vi "getProperty.vi"(8 "error in (no error)":errorcluster, 10 "Property Name in":string, 11 "IPropertyObject in":refnum<class "IPropertyObject.lvclass">) -> (0 "error out":errorcluster, 2 "Property out":refnum<class "IProperty.lvclass">, 3 "IPropertyObject out":refnum<class "IPropertyObject.lvclass">)   [LabVIEW 2022 SP3, in "openDAQ.lvlib" / "IBaseObject.lvlib" / "IPropertyObject.lvlib" / "IPropertyObject.lvclass"]
uses:
  <instrlib>/openDAQ/Public/Classes/IPropertyObject/IPropertyObject.lvclass
  <instrlib>/openDAQ/Public/Classes/IPropertyObject/IPropertyObject.lvclass/IPropertyObject.ctl
  <instrlib>/openDAQ/Public/Classes/daqCoreTypes/IString/IString.lvclass
  <instrlib>/openDAQ/Public/Classes/IProperty/IProperty.lvclass
  <instrlib>/openDAQ/Binaries/Windows/x86/copendaq32.dll
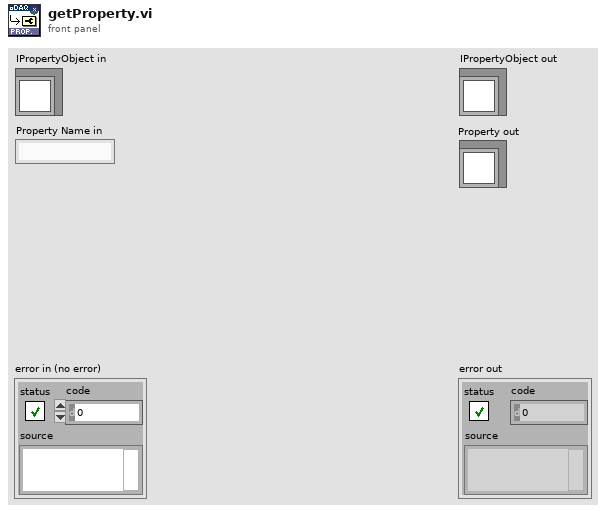
[diagram p1: front panel]
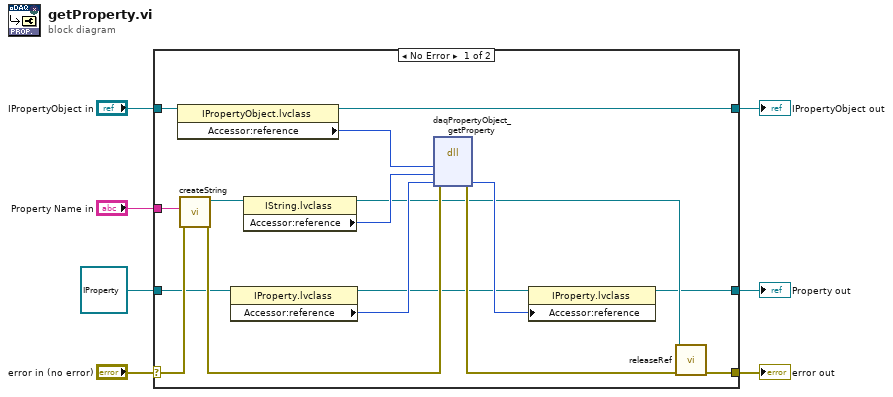
[diagram p0: block diagram]
diagram:
  n1 = case shown="No Error" "error in (no error)" {
    selector: "error in (no error)" -> [w18 w26]
    tunnel: [w13 w26] -> w6
    tunnel: [w19 w25] -> w4
    tunnel: "IPropertyObject in" -> [w21 w25]
    tunnel: "Property Name in" -> [w16 _]
    tunnel: refnum<class "IProperty.lvclass"> refnum ("openDAQ.lvlib:IBaseObject.lvlib:IProperty.lvlib:IProperty.lvclass") -> [w10 w24]
    tunnel: [w8 w24] -> w1
    frame No Error {
      n2 = property class="IPropertyObject.lvclass"(reference=w21) -> (reference out=w19:refnum<class "IPropertyObject.lvclass">, "Accessor:reference"=w20:i64)  [unwired: 1 in, 1 out]
      n3 = call <instrlib>:"createString.vi"("error in (no error)"=w18, "String"=w16) -> ("error out"=w17:errorcluster, "IString out"=w15:refnum<class "IString.lvclass">)  [unwired: 8 in]
      n4 = property class="IProperty.lvclass"(reference=w10) -> (reference out=w9:refnum<class "IProperty.lvclass">, "Accessor:reference"=w22:i64)  [unwired: 1 in, 1 out]
      n5 = property class="IString.lvclass"(reference=w15) -> (reference out=w11:refnum<class "IString.lvclass">, "Accessor:reference"=w14:i64)  [unwired: 1 in, 1 out]
      n6 = dll-call lib="C:/Program Files (x86)/National Instruments/LabVIEW 2022/instr.lib/openDAQ/Binaries/Windows/x86/copendaq*.*" fn="daqPropertyObject_getProperty"(error in=w17, "propertyObject"=w20, "name"=w14, "hasProperty"=w22) -> (error out=w12:errorcluster, "hasProperty"=w23:i64)  [unwired: 5 in, 1 out]
      n7 = property class="IProperty.lvclass"(reference=w9, "Accessor:reference"=w23) -> (reference out=w8:refnum<class "IProperty.lvclass">)  [unwired: 1 in, 1 out]
      n8 = call-dynamic "releaseRef.vi"("error in (no error)"=w12, "IBaseObject in"=w11) -> ("error out"=w13:errorcluster)  [unwired: 9 in]
    }
    frame Error {
    }
  }
  "error out" <- w6
  "IPropertyObject out" <- w4
  "Property out" <- w1
